vi "NI.History (String).vi"(1 "value in":string) -> (0 "Stop?":bool)   [LabVIEW 2020]
doc: "Displays the value of the 32-bit signed integer numeric control and allows conditional breakpoints."
uses:
  <vilib>/Utility/miscctls.llb/LVRowAndColumnUnsignedTypeDef.ctl
panel:
  out "History":i32(listbox)=-1
  out "Hex":string
  out "\\ Codes":string
  in  "Display Style":u16(ring) items=["Normal Display", "'\\' Codes Display", "Hex Display"]
  in  "Ignore Empty?":bool
  in  "reset":bool
  # "* Changes to these options take effect the next time the probe runs."
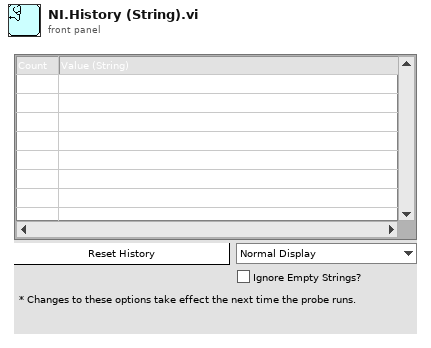
[diagram p1: front panel]
types:
  T1 = typedef "LVRowAndColumnUnsignedTypeDef.ctl" = cluster{"Row":u32, "Column":u32}
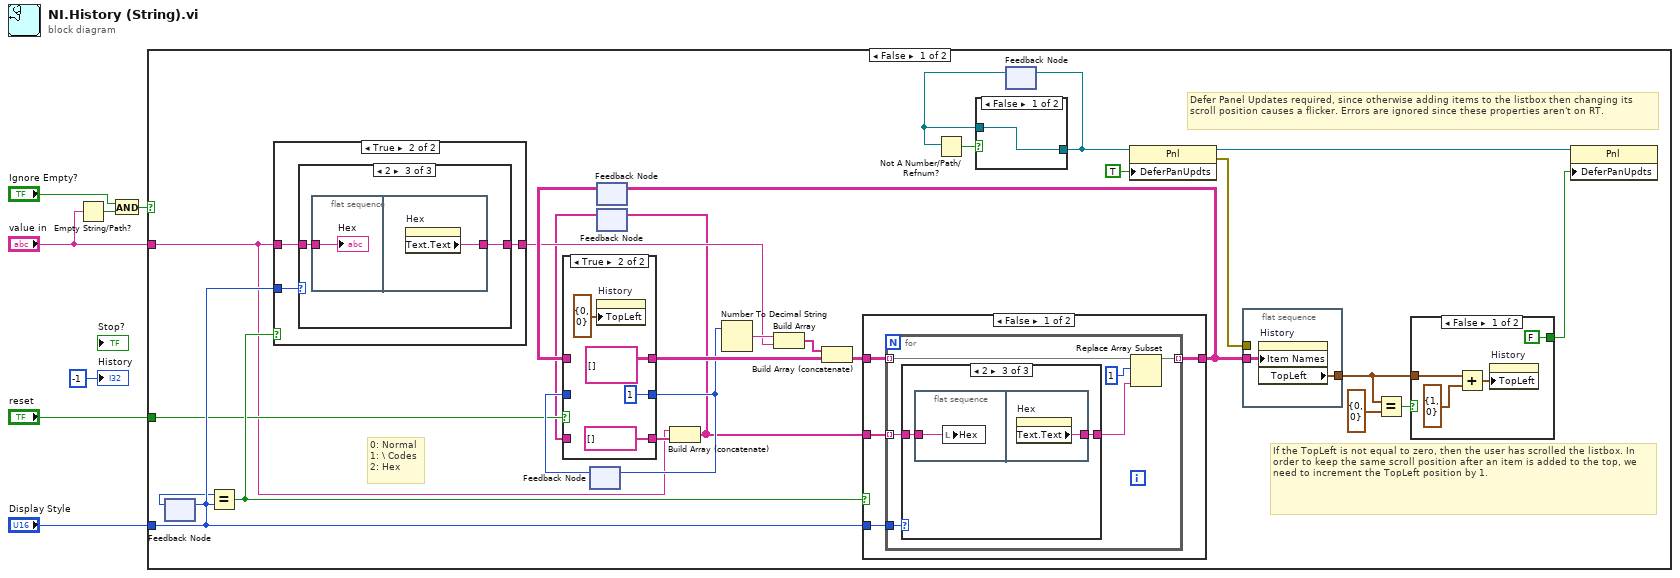
[diagram p0: block diagram]
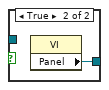
[diagram p3: hidden frame]
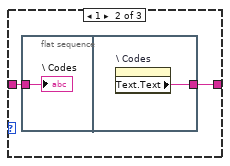
[diagram p6: hidden frame]
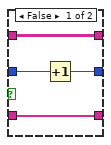
[diagram p7: hidden frame]
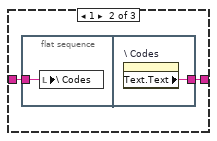
[diagram p9: hidden frame]
diagram:
  n1 = Empty String/Path?(string/path="value in") -> (empty?=w4:bool)
  n2 = And(x="Ignore Empty?", y=w4) -> (x .and. y?=w2:bool)
  n3 = case shown="False" w2 {
    tunnel: "reset" -> [w22 _]
    tunnel: "value in" -> [w19 _]
    tunnel: "Display Style" -> [w24 _]
    frame False {
      # "If the TopLeft is not equal to zero, then the user has scrolled the listbox. In order to keep the same scroll position after an item is added to the top, we need to increment the TopLeft position by 1."
      # "Defer Panel Updates required, since otherwise adding items to the listbox then changing its scroll position causes a flicker. Errors are ignored since these properties aren't on RT."
      # "0: Normal\n1: \\ Codes\n2: Hex"
      n4 = feedback #1() -> (w23:u16)  [unwired: 1 in]
      n5 = feedback-in #1(w24) -> ()
      n6 = Equal?(x=w23, y=w24) -> (x = y?=w26:bool)
      n7 = case shown="True" w26 {
        tunnel: w19 -> [w43 w45]
        tunnel: [w43 w44] -> w25
        tunnel: w24 -> [_ w46]
        frame False {
          # "Don't bother doing the formatting here when the style changes, as the whole list is going to get reformatted later."
        }
        frame True {
          n8 = case shown="2" w46 {
            tunnel: w45 -> [w47 w49 w53]
            tunnel: [w47 w48 w52] -> w44
            frame Default {
            }
            frame 1 {
              n9 = flat-sequence {
                tunnel: w49 -> [w50]
                tunnel: [w51] -> w48
                frame #0 {
                  "\\ Codes" <- w50
                }
                frame #1 {
                  n10 = property on="\\ Codes" class="Str"() -> ("Text.Text"=w51:string)  [unwired: 2 in, 2 out]
                }
              }
            }
            frame 2 {
              n11 = flat-sequence {
                tunnel: w53 -> [w54]
                tunnel: [w55] -> w52
                frame #0 {
                  "Hex" <- w54
                }
                frame #1 {
                  n12 = property on="Hex" class="Str"() -> ("Text.Text"=w55:string)  [unwired: 2 in, 2 out]
                }
              }
            }
          }
        }
      }
      n13 = feedback #2() -> (w30:i32)  [unwired: 1 in]
      n14 = feedback #3() -> (w29:string[][])  [unwired: 1 in]
      n15 = feedback #4() -> (w20:string[])  [unwired: 1 in]
      n16 = case shown="True" w22 {
        tunnel: w29 -> [w59 _]
        tunnel: w30 -> [w58 _]
        tunnel: [w59 string[][] []] -> w34
        tunnel: [w57 1] -> w31
        tunnel: [w56 string[] []] -> w21
        tunnel: w20 -> [w56 _]
        frame False {
          n17 = Increment(x=w58) -> (x+1=w57:i32)
        }
        frame True {
          n18 = property on="History" class="MCListbox (strict)"("TopLeft"=T1 {"Row"=0, "Column"=0} ("Top Left Visible Cell")) -> ()  [unwired: 2 in, 2 out]
        }
      }
      n19 = feedback-in #2(w31) -> ()
      n20 = Build Array (concatenate)(w19, w21) -> (w18:string[])
      n21 = feedback-in #4(w18) -> ()
      n22 = Number To Decimal String(number=w31) -> (decimal integer string=w32:string)  [unwired: 1 in]
      n23 = Build Array(w32, w25) -> (w33:string[])
      n24 = Build Array (concatenate)(w33, w34) -> (w27:string[][])
      n25 = case shown="False" w26 {
        tunnel: [w66 w83] -> w28
        tunnel: w27 -> [w67 w83]
        tunnel: w24 -> [w65 _]
        tunnel: w18 -> [w64 _]
        frame False {
          n26 = for {
            tunnel: w67 -> [w73] mode=indexing
            tunnel: [w72] -> w66 mode=indexing
            tunnel: w65 -> [w70]
            tunnel: w64 -> [w68] mode=indexing
            n27 = case shown="2" w70 {
              tunnel: w68 -> [w74 w76 w80]
              tunnel: [w74 w75 w79] -> w69
              frame 0, Default {
              }
              frame 1 {
                n28 = flat-sequence {
                  tunnel: w76 -> [w77]
                  tunnel: [w78] -> w75
                  frame #0 {
                    n29 = local write "\\ Codes"(w77) -> ()
                  }
                  frame #1 {
                    n30 = property on="\\ Codes" class="Str"() -> ("Text.Text"=w78:string)  [unwired: 2 in, 2 out]
                  }
                }
              }
              frame 2 {
                n31 = flat-sequence {
                  tunnel: w80 -> [w81]
                  tunnel: [w82] -> w79
                  frame #0 {
                    n32 = local write "Hex"(w81) -> ()
                  }
                  frame #1 {
                    n33 = property on="Hex" class="Str"() -> ("Text.Text"=w82:string)  [unwired: 2 in, 2 out]
                  }
                }
              }
            }
            n34 = Replace Array Subset(array=w73, new element=w69, index=1) -> (w72:string[])
          }
        }
        frame True {
        }
      }
      n35 = feedback-in #3(w28) -> ()
      n36 = feedback #5() -> (w14:refnum<vi>)  [unwired: 1 in]
      n37 = Not A Number/Path/Refnum?(number/path/refnum=w14) -> (NaN/Path/Refnum?=w15:bool)
      n38 = case shown="False" w15 {
        tunnel: [w41 w42] -> w16
        tunnel: w14 -> [w41 _]
        frame False {
        }
        frame True {
          n39 = property class="VI"() -> ("Panel"=w42:refnum<vi>)  [unwired: 2 in, 2 out]
        }
      }
      n40 = feedback-in #5(w16) -> ()
      n41 = property class="Pnl"(reference=w16, "DeferPanUpdts"=TRUE ("Defer Panel Updates")) -> (reference out=w13:refnum<vi>, error out=w12:errorcluster)  [unwired: 1 in]
      n42 = flat-sequence {
        tunnel: w28 -> [w36]
        tunnel: w12 -> [_]
        tunnel: [w35] -> w9
        frame #0 {
          n43 = property on="History" class="MCListbox (strict)"("Item Names"=w36) -> ("TopLeft"=w35:T1)  [unwired: 2 in, 2 out]
        }
      }
      n44 = Equal?(x=w9, y=T1 {"Row"=0, "Column"=0} ("Top Left Visible Cell")) -> (x = y?=w10:bool)
      n45 = case shown="False" w10 {
        tunnel: w9 -> [w40 _]
        tunnel: [FALSE ("Defer Panel Updates") _] -> w8
        frame False {
          n46 = Add(x=w40, y=T1 {"Row"=1, "Column"=0}) -> (x+y=w38:T1)
          n47 = property on="History" class="MCListbox (strict)"("TopLeft"=w38) -> ()  [unwired: 2 in, 2 out]
        }
        frame True {
        }
      }
      n48 = property class="Pnl"(reference=w13, "DeferPanUpdts"=w8) -> ()  [unwired: 1 in, 2 out]
    }
    frame True {
    }
  }
  "History" <- -1 ("History of Values")
